vi "GyroAccel - Initialise GyroAccel.vi"(8 "error in (no error)":errorcluster) -> (0 "error out":errorcluster, 1 "Gyro Self-Test (Disabled)":u8[](array[numeric]), 2 "Who Am I":u8[](array[numeric]))   [LabVIEW 2021]
uses:
  <vilib>/myRIO/Instrument Drivers/Onboard IO/I2C/typedefs/I2C User Configuration.ctl
  <vilib>/myRIO/Instrument Drivers/Onboard IO/I2C/typedefs/I2C Transfer Rate.ctl
  <vilib>/myRIO/Instrument Drivers/Onboard IO/I2C/typedefs/I2C Reference.ctl
  <vilib>/myRIO/Common/Instrument Driver Framework/Utilities/typedefs/myRIO Generic Hardware Reference.ctl
  <vilib>/myRIO/Common/Instrument Driver Framework/Utilities/typedefs/Hardware Version Enum.ctl
  <vilib>/myRIO/Common/Instrument Driver Framework/Utilities/typedefs/myRIO v1.0 Reference.ctl
  <vilib>/myRIO/Common/Instrument Driver Framework/Utilities/typedefs/Generic FPGA Reference.ctl
  <vilib>/myRIO/Common/Instrument Driver Framework/myRIO v1.0/I2C/typedefs/I2C Channels Enum.ctl
  <vilib>/myRIO/Instrument Drivers/Onboard IO/I2C/typedefs/I2C Configuration.ctl
  <vilib>/userDefined/High Color/nirio_resource_hc.ctl
  <vilib>/myRIO/Common/Instrument Driver Framework/Utilities/vis/Is FPGA Ref Available.vi
  <vilib>/myRIO/Common/Instrument Driver Framework/myRIO v1.0/I2C/vis/myRIO v1.1 Open I2C.vi
  <vilib>/myRIO/Instrument Drivers/Onboard IO/I2C/vis/Configure.vi
  <vilib>/myRIO/Instrument Drivers/Onboard IO/I2C/vis/Write Read.vi
  <vilib>/myRIO/Instrument Drivers/Onboard IO/I2C/vis/Write.vi
  <vilib>/myRIO/Common/Instrument Driver Framework/Utilities/vis/Validate Channels.vi
  <vilib>/myRIO/Common/Instrument Driver Framework/myRIO v1.0/I2C/vis/myRIO v1.0 Reserve I2C.vi
  <vilib>/myRIO/Common/Instrument Driver Framework/myRIO v1.0/I2C/vis/myRIO v1.0 Build MUX Configuration I2C.vi
  <vilib>/myRIO/Common/Instrument Driver Framework/myRIO v1.0/Resource Manager/vis/myRIO v1.0 Reserve Channel List.vi
  <vilib>/myRIO/Common/Instrument Driver Framework/myRIO v1.0/Resource Manager/vis/myRIO v1.0 Create Configuration List.vi
  <vilib>/myRIO/Common/Instrument Driver Framework/myRIO v1.0/Resource Manager/vis/myRIO v1.0 Reserve Channel.vi
  <vilib>/myRIO/Common/Instrument Driver Framework/myRIO v1.0/Resource Manager/vis/myRIO v1.0 Unreserve Channel.vi
  <vilib>/myRIO/Common/Instrument Driver Framework/myRIO v1.0/Resource Manager/vis/myRIO v1.0 Build Mutex Name.vi
  <vilib>/Utility/VariantDataType/GetNumericInfo.vi
  <vilib>/Utility/error.llb/Error Cluster From Error Code.vi
  <vilib>/myRIO/Common/Instrument Driver Framework/myRIO v1.0/myRIO v1.1 Open.vi
  <vilib>/myRIO/Common/Instrument Driver Framework/Utilities/vis/IO Manager.vi
  <vilib>/myRIO/Common/Instrument Driver Framework/Utilities/vis/Configuration Manager.vi
  <vilib>/myRIO/Common/Instrument Driver Framework/myRIO v1.0/Resource Manager/vis/myRIO v1.0 Configure IO.vi
  <vilib>/myRIO/Common/Instrument Driver Framework/myRIO v1.0/myRIO v1.0 Close.vi
  <vilib>/myRIO/Common/Instrument Driver Framework/myRIO v1.0/I2C/vis/myRIO v1.0 Configure I2C.vi
  <vilib>/myRIO/Common/Instrument Driver Framework/myRIO v1.0/I2C/vis/myRIO v1.0 Write I2C.vi
  <vilib>/myRIO/Common/Instrument Driver Framework/myRIO v1.0/I2C/vis/myRIO v1.0 Read I2C.vi
  <vilib>/myRIO/Express VI/Onboard IO/I2C/I2C Express VI.xnode
  <vilib>/myRIO/Instrument Drivers/Onboard IO/I2C/vis/myRIO I2C Open.xnode
  <vilib>/myRIO/Instrument Drivers/Onboard IO/I2C/I2C.lvlib
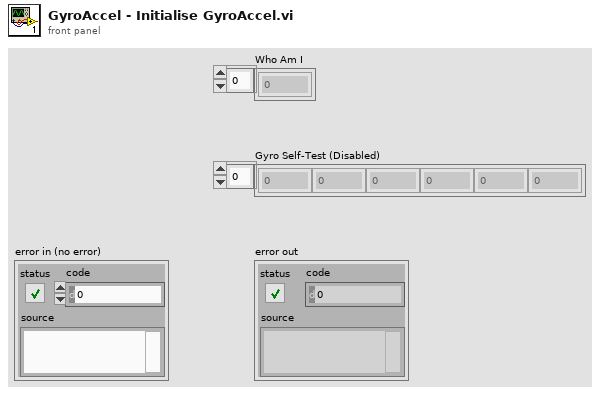
[diagram p1: front panel]
types:
  T1 = typedef "I2C.lvlib/I2C Reference.ctl" = cluster{"myRIO Reference":T2, "I2C Channels Enum":T6, "I2C Configuration":T7}
  T2 = typedef "myRIO Generic Hardware Reference.ctl" = cluster{"myRIO Model":T3, "myRIO Hardware Reference":T4}
  T3 = typedef "Hardware Version Enum.ctl" = enum16{"Unknown", "myRIO-1900", "myRIO-1950", "roboRIO", "NI ELVIS RIO CM", "ELVIS III"}
  T4 = typedef "myRIO v1.0 Reference.ctl" = cluster{"Generic FPGA Reference":T5, "Allow multiple opens":bool}
  T5 = typedef "Generic FPGA Reference.ctl" = refnum<k20>
  T6 = typedef "I2C Channels Enum.ctl" = enum16{"Not Connected", "A/I2C", "B/I2C", "I2C/I2C"}
  T7 = typedef "I2C.lvlib/I2C Configuration.ctl" = cluster{"I2C Transfer Rate":T8}
  T8 = typedef "I2C.lvlib/I2C Transfer Rate.ctl" = enum16{"Standard mode (100 kbps)", "Fast mode (400 kbps)"}
  T9 = typedef "I2C.lvlib/I2C User Configuration.ctl" = cluster{"I2C Transfer Rate":T8}
  T10 = typedef "nirio_resource_hc.ctl" = tag
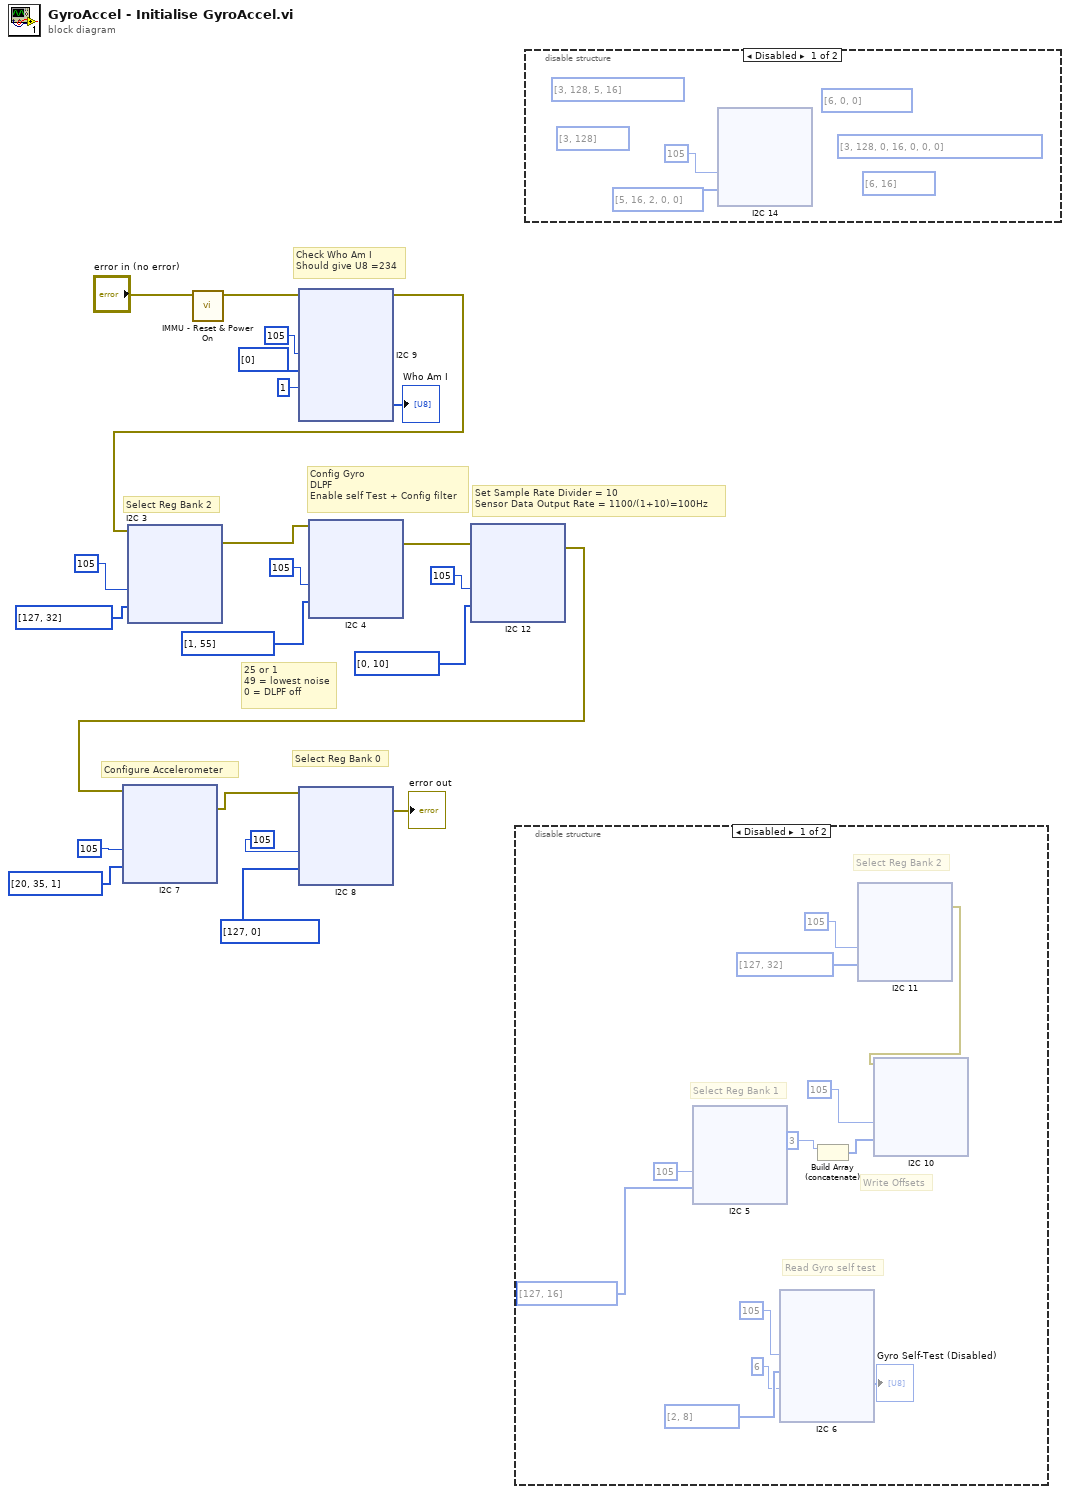
[diagram p0: block diagram]
diagram:
  # "Set Sample Rate Divider = 10\nSensor Data Output Rate = 1100/(1+10)=100Hz"
  # "Check Who Am I \nShould give U8 =234"
  # "25 or 1 \n49 = lowest noise\n0 = DLPF off"
  # "Configure Accelerometer"
  # "Select Reg Bank 0"
  # "Config Gyro\nDLPF\nEnable self Test + Config filter"
  # "Select Reg Bank 2"
  n1 = call "IMMU - Reset & Power On.vi"("error in (no error)"="error in (no error)") -> ("error out"=w2:errorcluster)  [unwired: 10 in]
  n2 = xnode "I2C 9"("Slave Address (7-bit)"=u8 105, "Bytes to Write"=u8[] [0], "Byte Count"=u32 1, "error in (no error)"=w2) -> ("Bytes Read"=→"Who Am I":u8[], "error out"=w11:errorcluster)
  n3 = xnode "I2C 3"("Slave Address (7-bit)"=u8 105, "Bytes to Write"=u8[] [127, 32], "error in (no error)"=w11) -> ("error out"=w4:errorcluster)
  n4 = xnode "I2C 4"("Slave Address (7-bit)"=u8 105, "Bytes to Write"=u8[] [1, 55], "error in (no error)"=w4) -> ("error out"=w20:errorcluster)
  n5 = xnode "I2C 12"("Slave Address (7-bit)"=u8 105, "Bytes to Write"=u8[] [0, 10], "error in (no error)"=w20) -> ("error out"=w19:errorcluster)
  n6 = xnode "I2C 7"("Slave Address (7-bit)"=u8 105, "Bytes to Write"=u8[] [20, 35, 1], "error in (no error)"=w19) -> ("error out"=w22:errorcluster)
  n7 = xnode "I2C 8"("Slave Address (7-bit)"=u8 105, "Bytes to Write"=u8[] [127, 0], "error in (no error)"=w22) -> ("error out"=→"error out":errorcluster)
  n8 = disable-structure shown="Disabled" {
    frame Disabled {
      # "Select Reg Bank 1"
      # "Read Gyro self test"
      # "Write Offsets"
      # "Select Reg Bank 2"
      n9 = xnode "I2C 5"("Slave Address (7-bit)"=u8 105, "Bytes to Write"=u8[] [127, 16]) -> ()  [unwired: 1 in, 1 out]
      n10 = xnode "I2C 6"("Slave Address (7-bit)"=u8 105, "Bytes to Write"=u8[] [2, 8], "Byte Count"=u32 6) -> ("Bytes Read"=→"Gyro Self-Test (Disabled)":u8[])  [unwired: 1 in, 1 out]
      n11 = Build Array (concatenate)(u8 3) -> (w29:u8[])  [unwired: 1 in]
      n12 = xnode "I2C 11"("Slave Address (7-bit)"=u8 105, "Bytes to Write"=u8[] [127, 32]) -> ("error out"=w32:errorcluster)  [unwired: 1 in]
      n13 = xnode "I2C 10"("Slave Address (7-bit)"=u8 105, "Bytes to Write"=w29, "error in (no error)"=w32) -> ()  [unwired: 1 out]
    }
    frame Enabled {
    }
  }
  n14 = disable-structure shown="Disabled" {
    frame Disabled {
      (unwired) u8[] [6, 16]
      (unwired) u8[] [3, 128]
      (unwired) u8[] [3, 128, 0, 16, 0, 0, 0]
      (unwired) u8[] [3, 128, 5, 16]
      (unwired) u8[] [6, 0, 0]
      n15 = xnode "I2C 14"("Slave Address (7-bit)"=u8 105, "Bytes to Write"=u8[] [5, 16, 2, 0, 0]) -> ()  [unwired: 1 in, 1 out]
    }
    frame Enabled {
    }
  }
